vi "DQMH Prepare (Cloneable).vi"(7 "Path to module directory":path, 8 "error in (no error)":errorcluster, 10 "Module ID":i32, 11 "Application reference":refnum<vi>) -> (0 "error out":errorcluster)   [LabVIEW 2014, in "hse-dqmh-dynamicrequesters.lvlib"]
doc: "Calls the \"Prepare\" request VI of the module in <b>path</b>\n\n____\nHAMPEL SOFTWARE ENGINEERING v0.7.0 (2018-07-16 18:12)"
uses:
  hse-dqmh-dynamicrequesters.lvlib
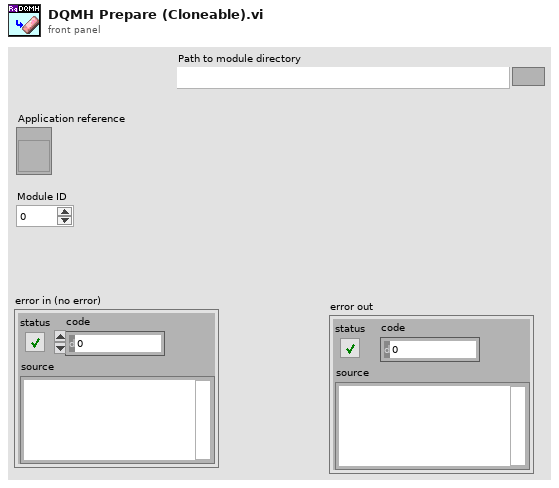
[diagram p1: front panel]
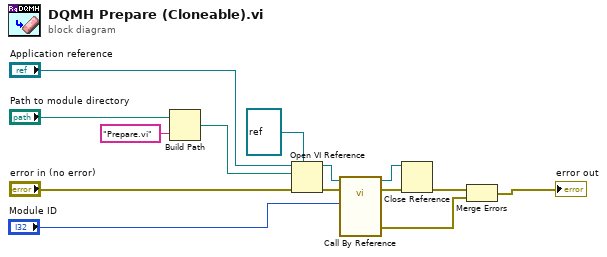
[diagram p0: block diagram]
diagram:
  n1 = Build Path(base path="Path to module directory", name or relative path="Prepare.vi") -> (appended path=w3:path)
  n2 = Open VI Reference(type specifier VI Refnum (for type only)=refnum<vi> refnum, application reference (local)="Application reference", vi path=w3, error in (no error)="error in (no error)") -> (vi reference=w4:refnum<vi>, error out=w5:errorcluster)  [unwired: 2 in]
  n3 = call-by-ref "?"(reference=w4, error in=w5, "Module ID"="Module ID") -> (reference out=w10:refnum<vi>, error out=w9:errorcluster, 0:"error out"=w12:errorcluster)  [unwired: 10 in]
  n4 = Close Reference(reference=w10, error in (no error)=w9) -> (error out=w8:errorcluster)
  n5 = Merge Errors(w8, w12) -> (→"error out":errorcluster)
